vi "Fetch Multi Eval Meas List Segment SEM Detected Allocation Results.vi"(7 "Segment (1)":T3=1, 8 "error in (no error)":errorcluster, 10 "Instance (1)":T4=1, 11 "VISA resource name":refnum<visa-resource-name>) -> (0 "error out":errorcluster, 1 "Detected Allocation":T2, 2 "Reliability Results":T1, 3 "VISA resource name out":refnum<visa-resource-name>)   [LabVIEW 2015, in "Rohde&Schwarz CMXP NR FR2 Measurement.lvlib"]
doc: "Returns the detected allocation for segment <no> in list mode.\n\nAttribute:\nRSCMXPNRFR2M_ATTR_FETCH_MULTI_EVAL_MEASUREMENT_LIST_SEGMENT_SEM_DETECTED_ALLOCATION_RESULTS\n\nRemote-control command:\nFETCh:NRMMw:MEAS<i>:MEValuation:LIST:SEGMent<no>:SEMask:DALLocation?"
uses:
  <instrlib>/Rohde&Schwarz CMXP NR FR2 Measurement/Rohde&Schwarz CMXP NR FR2 Measurement.lvlib
  <instrlib>/Rohde&Schwarz CMXP NR FR2 Measurement/Private/_Instance.ctl
  <instrlib>/Rohde&Schwarz CMXP NR FR2 Measurement/Private/_Segment.ctl
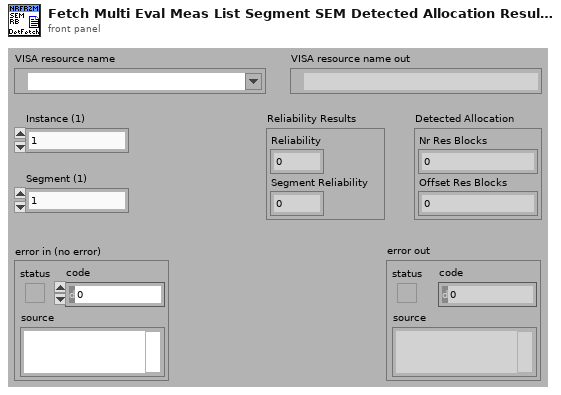
[diagram p1: front panel]
types:
  T1 = cluster{"Reliability":i32, "Segment Reliability":i32}
  T2 = cluster{"Nr Res Blocks":i32, "Offset Res Blocks":i32}
  T3 = typedef "Rohde&Schwarz CMXP NR FR2 Measurement.lvlib/_Segment.ctl" = i32
  T4 = typedef "Rohde&Schwarz CMXP NR FR2 Measurement.lvlib/_Instance.ctl" = i32
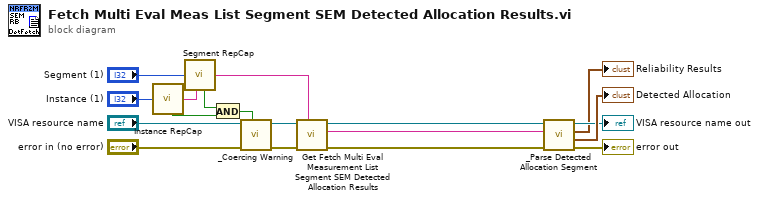
[diagram p0: block diagram]
diagram:
  n1 = call <instrlib>:"Instance RepCap.vi"("Instance In"="Instance (1)") -> ("In Range?"=w16:bool, "RepCap Identifier Out"=w1:string)  [unwired: 1 in]
  n2 = call <instrlib>:"Segment RepCap.vi"("Segment In"="Segment (1)", "RepCap String In (\"\")"=w1) -> ("In Range?"=w17:bool, "RepCap Identifier Out"=w10:string)
  n3 = And(x=w17, y=w16) -> (x .and. y?=w18:bool)
  n4 = call <instrlib>:"_Coercing Warning.vi"("In Range?"=w18, "error in (no error)"="error in (no error)", "VISA resource name"="VISA resource name") -> ("error out"=w11:errorcluster, "VISA resource name out"=w12:refnum<visa-resource-name>)  [unwired: 7 in]
  n5 = call "Get Fetch Multi Eval Measurement List Segment SEM Detected Allocation Results"("Repeated Capabilities"=w10, "error in (no error)"=w11, "instrument handle"=w12) -> ("error out"=w7:errorcluster, "Fetch Multi Eval Measurement List Segment SEM Detected Allocation Results"=w8:string, "instrument handle out"=w9:refnum<visa-resource-name>)  [unwired: 6 in]
  n6 = call <instrlib>:"_Parse Detected Allocation Segment.vi"("error in (no error)"=w7, "Input String"=w8, "VISA resource name"=w9) -> ("error out"=→"error out":errorcluster, "Detected Allocation"=→"Detected Allocation":T2, "Reliability Results"=→"Reliability Results":T1, "VISA resource name out"=→"VISA resource name out":refnum<visa-resource-name>)  [unwired: 5 in]
